vi "Error Handler - Message Handling Loop - Module.vi"(8 "DLL success":i32, 9 "error in (no error)":errorcluster, 11 "Shutdown?":bool=TRUE) -> (1 "dup error in":errorcluster, 2 "Shutdown!":bool, 4 "channel":T1)   [LabVIEW 2023, in "Message Queue Helper.lvlib"]
doc: "Process an error that occurred in the Message Handling Loop, either by ignoring it, or generating an \"Exit\" message."
uses:
  Message Queue Helper.lvlib
  <extravilib>/ChannelInstances/Messenger-t'Message Queue.lvlib-Message Cluster.ctl'/))Channel.ctl
  Message Cluster.ctl
  <extravilib>/ChannelInstances/Messenger-t'Message Queue.lvlib-Message Cluster.ctl'/Write.vi
  <extravilib>/ChannelInstances/Messenger-t'Message Queue.lvlib-Message Cluster.ctl'/Write With Abort.vi
  <extravilib>/ChannelInstances/Messenger-t'Message Queue.lvlib-Message Cluster.ctl'/Endpoint.vi
  Message Queue.lvlib
  <extravilib>/ChannelInstances/Messenger-t'Message Queue.lvlib-Message Cluster.ctl'.lvlib
panel:
  in  "Ignore Errors (Runtime)":i32[](array[numeric])
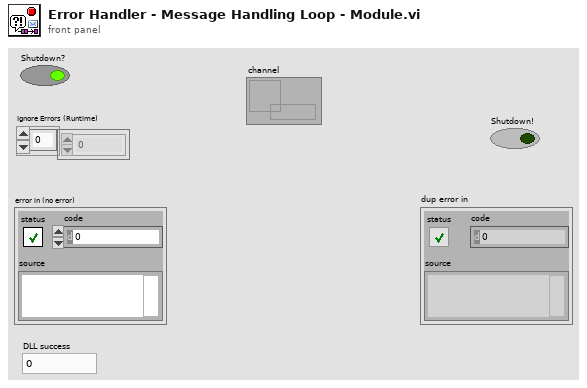
[diagram p1: front panel]
types:
  T1 = typedef "Messenger-t'Message Queue.lvlib-Message Cluster.ctl'.lvlib/))Channel.ctl" = refnum<queue>
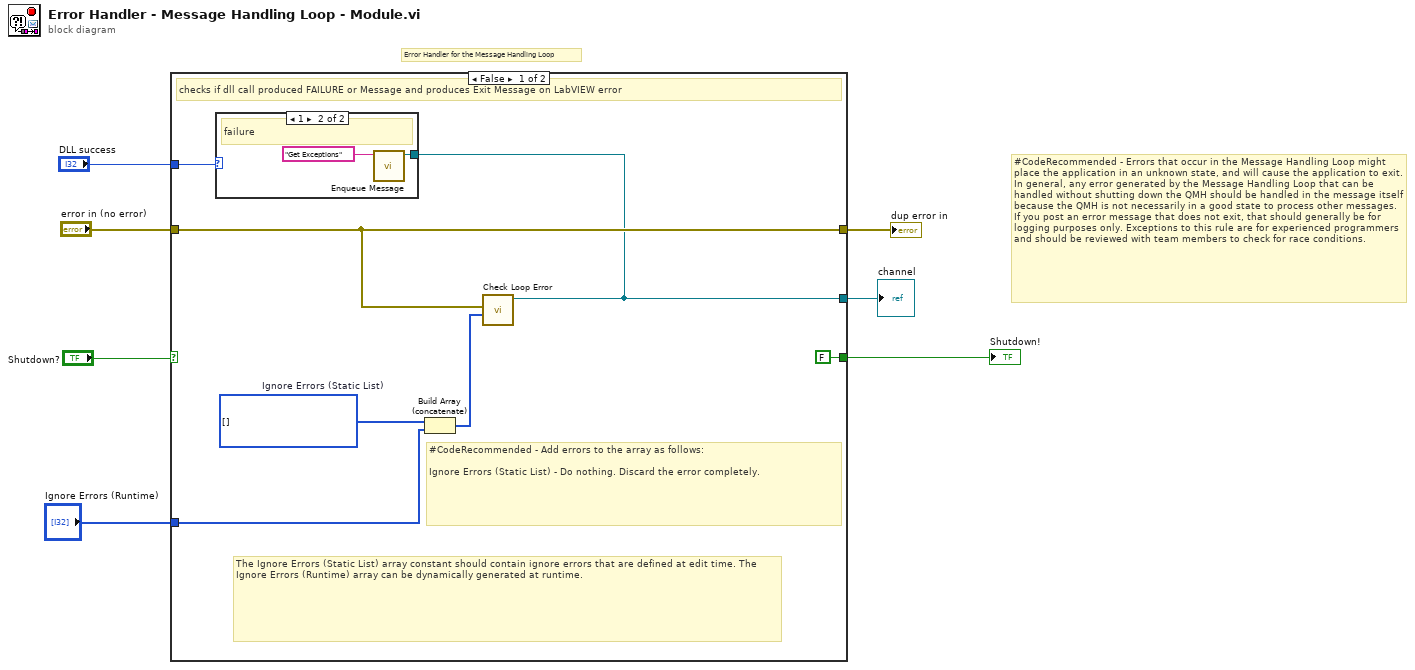
[diagram p0: block diagram]
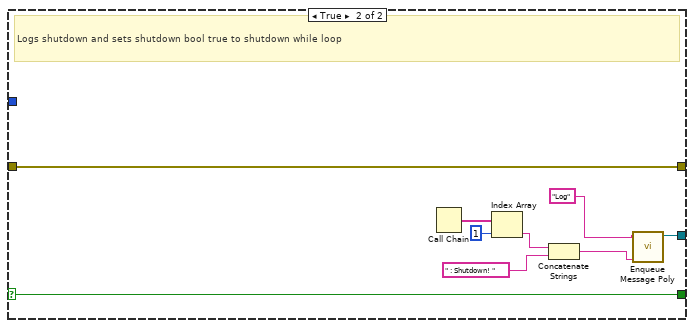
[diagram p3: hidden frame]
diagram:
  # "#CodeRecommended - Errors that occur in the Message Handling Loop might place the application in an unknown state, and will cause the application to exit. In general, any error generated by the Message Handling Loop that can be handled without shutting down the QMH should be handled in the message itself because the QMH is not necessarily in a good state to process other messages. If you post an error message that does not exit, that should generally be for logging purposes only. Exceptions to this rule are for experienced programmers and should be reviewed with team members to check for race conditions."
  # "Error Handler for the Message Handling Loop"
  n1 = case shown="False" "Shutdown?" {
    selector: "Shutdown?" -> [_ w25]
    tunnel: "error in (no error)" -> [w12 w19]
    tunnel: [w8 w23] -> w1
    tunnel: [w12 w19] -> w6
    tunnel: "Ignore Errors (Runtime)" -> [w11 _]
    tunnel: [FALSE w25] -> w3
    tunnel: "DLL success" -> [w9 _]
    frame False {
      w14 = i32[] []  # Ignore Errors (Static List)
      # "The Ignore Errors (Static List) array constant should contain ignore errors that are defined at edit time. The Ignore Errors (Runtime) array can be dynamically generated at runtime."
      # "#CodeRecommended - Add errors to the array as follows:\n\nIgnore Errors (Static List) - Do nothing. Discard the error completely."
      # "checks if dll call produced FAILURE or Message and produces Exit Message on LabVIEW error"
      n2 = case shown="1" w9 {
        tunnel: [_ w16] -> w8
        frame 0, Default {
          # "success"
        }
        frame 1 {
          # "failure"
          n3 = call "Enqueue Message.vi"("Message"="Get Exceptions") -> ("channel"=w16:T1)  [unwired: 10 in]
        }
      }
      n4 = Build Array (concatenate)(w14, w11) -> (w13:i32[])
      n5 = call "Check Loop Error.vi"("channel"=w8, "Ignore Errors"=w13, "error to process"=w12) -> ()  [unwired: 8 in, 1 out]
    }
    frame True {
      # "Logs shutdown and sets shutdown bool true to shutdown while loop"
      n6 = Call Chain() -> (call chain=w20:string[])
      n7 = Index Array(array=w20, index=1) -> (element=w21:string)
      n8 = Concatenate Strings(w21, " : Shutdown! " ("string")) -> (w17:string)
      n9 = call-poly "Enqueue Message Poly.vi"("Message Data"=w17, "Message"="Log" ("message")) -> ("channel"=w23:T1)  [unwired: 9 in]
    }
  }
  "dup error in" <- w6
  "Shutdown!" <- w3
  "channel" <- w1
